vi "Test.vi"() -> ()   [LabVIEW 2020, in "ABB-EL3000.lvlib" / "FID.lvlib" / "FID Kalibrierung.lvlib"]
uses:
  FID Kalibrierung.lvlib
  FID.lvlib
  Aktion STY_MES.ctl
panel:
  out "Zahlenanzeige.Text":string
  in  "Stopp":bool
  in  "Schreiben":bool
  in  "Enum":enum16{"Standby", "Messen"}(ring)
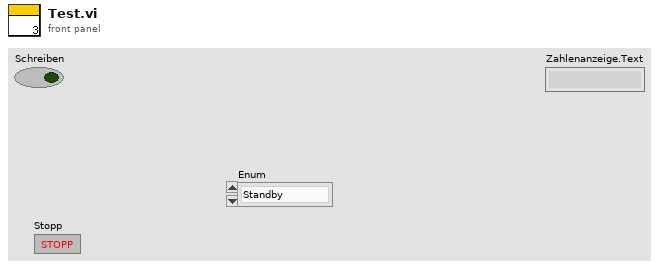
[diagram p1: front panel]
types:
  T1 = typedef "Aktion STY_MES.ctl" = enum16{"lesen", "setze STY", "setze MES", "MODBUS schreiben"}
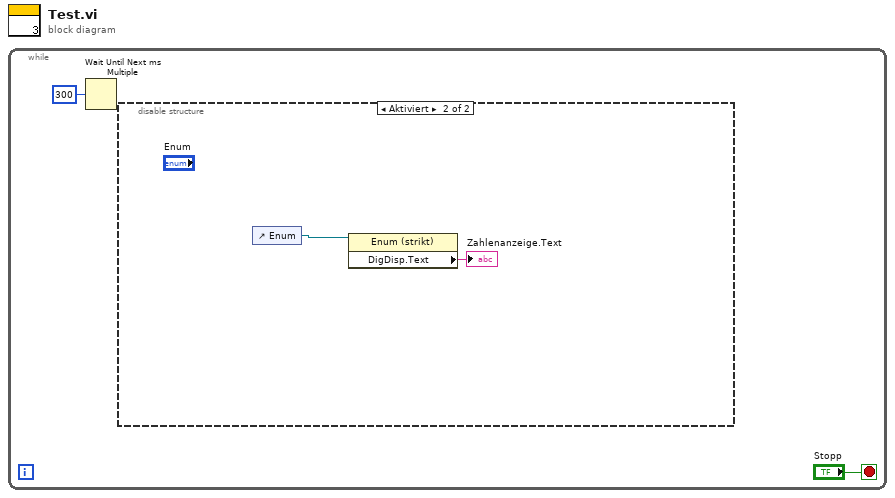
[diagram p0: block diagram]
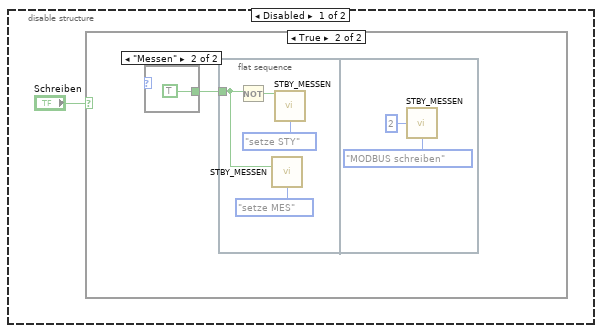
[diagram p2: hidden frame]
diagram:
  n1 = while {
    stop <- "Stopp" stop-if-true
    n2 = Wait Until Next ms Multiple(millisecond multiple=u32 300 ("Vielfache von ms")) -> ()  [unwired: 1 out]
    n3 = disable-structure shown="Aktiviert" {
      frame Disabled {
        n4 = case shown="True" "Schreiben" {
          frame False {
          }
          frame True {
            n5 = case shown="\"Messen\"" {
              selector: _ -> [_ _]
              tunnel: [_ TRUE] -> w4
              frame "Standby", Default {
              }
              frame "Messen" {
              }
            }
            n6 = flat-sequence {
              tunnel: w4 -> [w5]
              frame #0 {
                n7 = Not(x=w5) -> (.not. x?=w6:bool)
                n8 = call "STBY_MESSEN.vi"("Messen"=w5, "Aktion"=Aktion_STY_MES."setze MES") -> ()  [unwired: 10 in, 4 out]
                n9 = call "STBY_MESSEN.vi"("Standby"=w6, "Aktion"=Aktion_STY_MES."setze STY") -> ()  [unwired: 10 in, 4 out]
              }
              frame #1 {
                n10 = call "STBY_MESSEN.vi"("Case Nr."=2, "Aktion"=Aktion_STY_MES."MODBUS schreiben") -> ()  [unwired: 10 in, 4 out]
              }
            }
          }
        }
      }
      frame Enabled {
        n11 = control-ref of="Enum"() -> (w13:refnum<vi>)
        n12 = property class="Enum (strikt)"(reference=w13) -> ("DigDisp.Text"=→"Zahlenanzeige.Text":string)  [unwired: 1 in, 2 out]
      }
    }
  }
